vi "Encode-Decode test.vi"() -> ()   [LabVIEW 2026]
uses:
  Internal uServices/System uServices/Common GUI v3/Common GUI v3/Error Listbox Msg.ctl
  Internal uServices/System uServices/Common GUI v3/Common GUI v3/Error Listbox Msg Action.ctl
  Internal uServices/System uServices/Error Manager/Error Info.ctl
  Internal uServices/System uServices/TCP Writer/TCP Writer/TCP Message.ctl
  <vilib>/AdvancedString/1D String Array to Delimited String (string).vi
  Internal uServices/System uServices/TCP Writer/TCP Writer/TCP Writer.lvclass
  <userlib>/_OpenG.lib/lvdata/lvdata.llb/openg_variant.lvlib
  Internal uServices/System uServices/Error Manager/Error Manager.lvclass
  Internal uServices/System uServices/Common GUI v3/Common GUI v3/Common GUI v3.lvclass
panel:
  out "substring before match":string
  out "data":T1 {"Error Info"."Time Stamp" format="%<%x %.3X>T"}
  out "Array":i16[](array[numeric]) format="%x"
  out "Type Sting":string
  out "Data String":string
  out "type string":i16[](array[numeric])
  out "flattened string":string
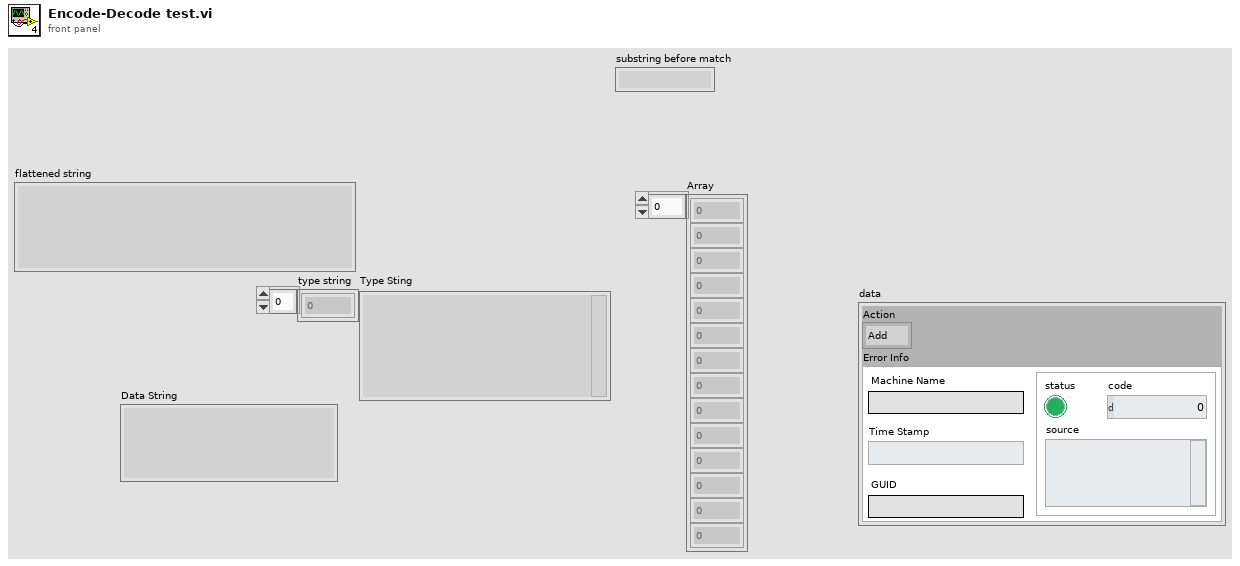
[diagram p1: front panel]
types:
  T1 = typedef "TALOS.lvlib/Common GUI v3.lvlib/Common GUI v3.lvclass/Error Listbox Msg.ctl" = cluster{"Action":T2, "Error Info":T3}
  T2 = typedef "TALOS.lvlib/Common GUI v3.lvlib/Common GUI v3.lvclass/Error Listbox Msg Action.ctl" = enum16{"Add", "Remove", "Clear"}
  T3 = typedef "TALOS.lvlib/Error Manager.lvlib/Error Manager.lvclass/Error Info.ctl" = cluster{"error out":errorcluster, "Time Stamp":timestamp, "Machine Name":string, "GUID":string}
  T4 = typedef "TALOS.lvlib/TCP Writer.lvlib/TCP Writer.lvclass/TCP Message.ctl" = cluster{"Type string":i16[], "Data string":string}
  T5 = cluster{"Target":string, "Topic":string, "Payload":cluster{"Strings":string[], cluster{cluster{"Error":cluster{"status":bool, "code":i32, "source":string, "Waveform":waveform(dbl)}}}[]}}
  T6 = cluster{"Target":string, "Topic":string, "Payload":variant}
  T7 = typedef "openg_variant.lvlib/Type Descriptor__ogtk.ctl" = i16[]
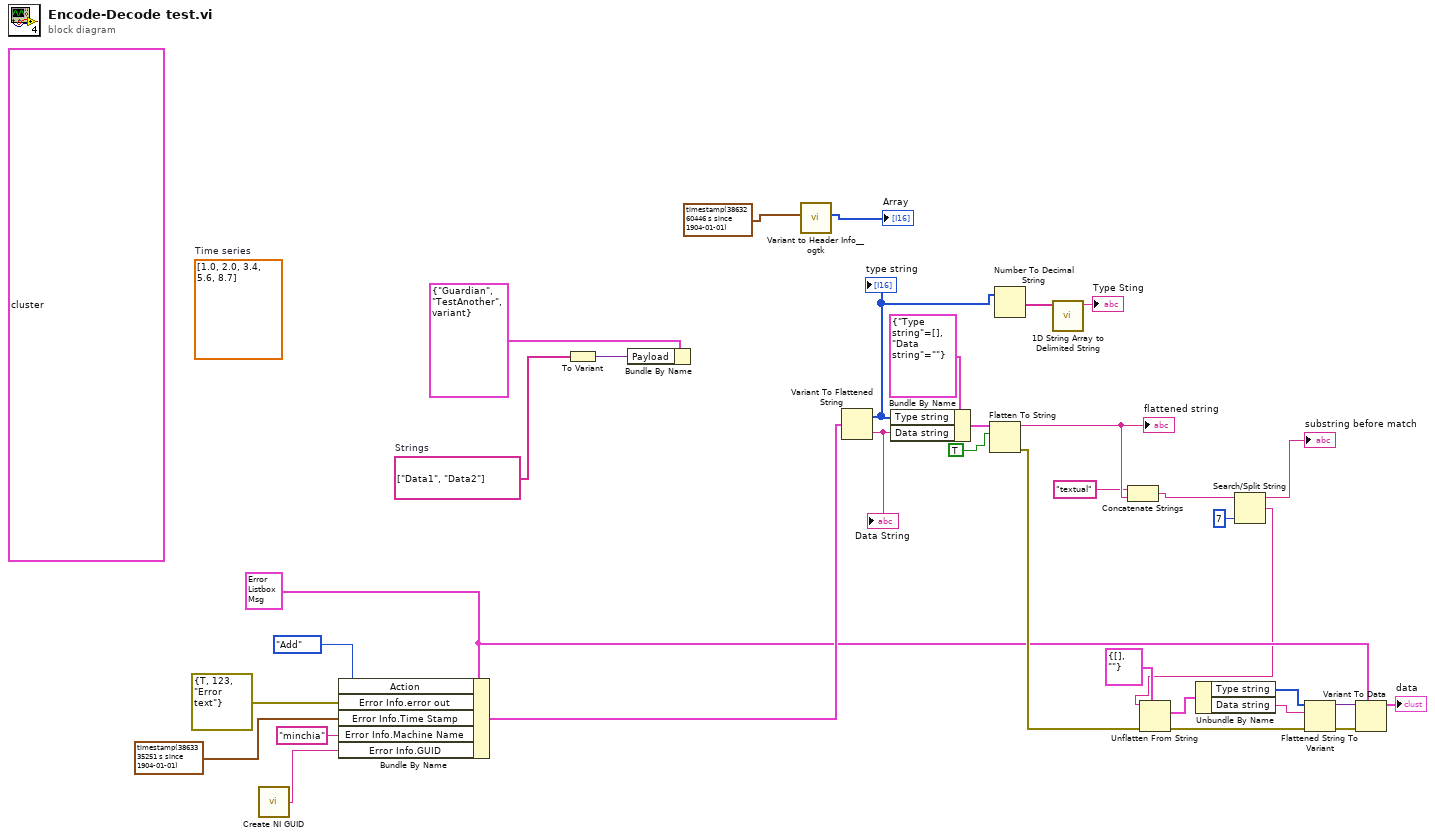
[diagram p0: block diagram]
diagram:
  w8 = T1 {"Action"=enum."Add", "Error Info"={"error out"={"status"=FALSE, "code"=0, "source"=""}, "Time Stamp"=timestamp(0 s since 1904-01-01), "Machine Name"="", "GUID"=""}} ("Error Listbox Msg")
  w25 = string[] ["Data1", "Data2"]  # Strings
  (unwired) T5 {"Target"="Guardian", "Topic"="TestAnother", "Payload"={"Strings"=["Data1", "Data2"], [{{"Error"={"status"=TRUE, "code"=123, "source"="Error text", "Waveform"={"t0"=timestamp(3863333701.5438056 s since 1904-01-01), "dt"=1.0, "Y"=[1.0]}}}}, {{"Error"={"status"=TRUE, "code"=2, "source"="Error text", "Waveform"={"t0"=timestamp(3479372122.009291 s since 1904-01-01), "dt"=1.0, "Y"=[5.0]}}}}]}}
  (unwired) dbl[] [1.0, 2.0, 3.4, 5.6, 8.7]  # Time series
  n1 = call <vilib>:"Create NI GUID.vi"() -> ("NI GUID"=w19:string)
  n2 = Bundle By Name(cluster=w8, "Action"=Error_Listbox_Msg_Action."Add", "Error Info.error out"=errorcluster {"status"=TRUE, "code"=123, "source"="Error text"}, "Error Info.Time Stamp"=timestamp(3863335251.141723 s since 1904-01-01), "Error Info.Machine Name"="minchia", "Error Info.GUID"=w19) -> (w18:T1)
  n3 = To Variant(anything=w25) -> (Variant=w24:variant)
  n4 = Bundle By Name(cluster=T6 {"Target"="Guardian", "Topic"="TestAnother", "Payload"=variant}, "Payload"=w24) -> ()  [unwired: 1 out]
  n5 = call <userlib>:"Variant to Header Info__ogtk.vi"("Variant"=timestamp(3863260446.7735906 s since 1904-01-01)) -> ("Type Descriptor"=→"Array":T7)  [unwired: 3 in, 2 out]
  n6 = Variant To Flattened String(Variant=w18) -> (data string=w32:string, 1:w31:i16[])
  "type string" <- w31
  "Data String" <- w32
  n7 = Bundle By Name(cluster=T4 {"Type string"=[], "Data string"=""}, "Type string"=w31, "Data string"=w32) -> (w34:T4)
  n8 = Flatten To String(anything=w34, prepend array or string size? (T)=TRUE) -> (data string=w6:string, error out=w11:errorcluster)  [unwired: 2 in, 1 out]
  "flattened string" <- w6
  n9 = Number To Decimal String(number=w31) -> (decimal integer string=w30:string[])  [unwired: 1 in]
  n10 = call-poly <vilib>:"1D String Array to Delimited String.vi"("string array"=w30) -> ("delimited string"=→"Type Sting":string)  [unwired: 10 in]
  n11 = Concatenate Strings("textual" ("string"), w6) -> (w5:string)
  n12 = Search/Split String(string=w5, offset (0)=7) -> (substring before match=→"substring before match":string, match + rest of string=w1:string)  [unwired: 1 in, 1 out]
  n13 = Unflatten From String(type=T4 {"Type string"=[], "Data string"=""}, binary string=w1, error in (no error)=w11) -> (value=w16:T4, error out=w17:errorcluster)  [unwired: 2 in, 1 out]
  n14 = Unbundle By Name(w16) -> ("Type string"=w12:i16[], "Data string"=w13:string)
  n15 = Flattened String To Variant(4:w17, 6:w13, 7:w12) -> (0:w15:errorcluster, 3:w14:variant)
  n16 = Variant To Data(error in=w15, type=w8, Variant=w14) -> (data=→"data":T1)  [unwired: 1 out]
